vi "Start Print.vi"(8 "error in (no error)":errorcluster, 11 "Feeder Actor.lvlib:Feeder.lvclass":refnum<class "Feeder.lvclass">) -> (0 "error out":errorcluster, 3 "Feeder Actor.lvlib:Feeder.lvclass":refnum<class "Feeder.lvclass">)   [LabVIEW 2018, in "Feeder Actor.lvlib" / "Feeder.lvclass"]
uses:
  Feeder.lvclass
  Feeder.lvclass/Feeder.ctl
  Solenoid Messages/Set Solonoid Msg/Set Solonoid Msg.lvclass/Set Solonoid Msg.ctl
  <vilib>/ActorFramework/Message Enqueuer/Message Enqueuer.lvclass/Message Enqueuer.ctl
  <vilib>/ActorFramework/Message Enqueuer/Enqueue.vi
  Solenoid Messages/Set Solonoid Msg/Set Solonoid Msg.lvclass
  C:/Program Files/National Instruments/LabVIEW 2018/vi.lib/ActorFramework/Message/Message.lvclass
  <vilib>/ActorFramework/Message Priority Queue/Priority Enqueue.vi
  Mixer Messages/Mixer Print Msg/Mixer Print Msg.lvclass
  Screw Messages/Screw Print Msg/Screw Print Msg.lvclass
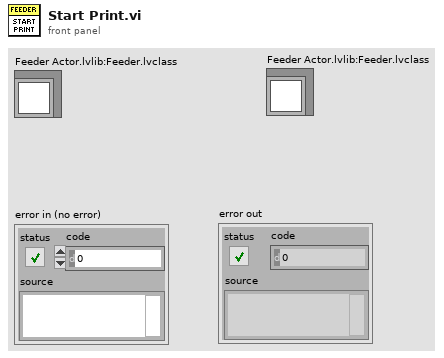
[diagram p1: front panel]
types:
  T1 = enum8{"Enabled", "Disabled", "Disabled and Grayed Out"}
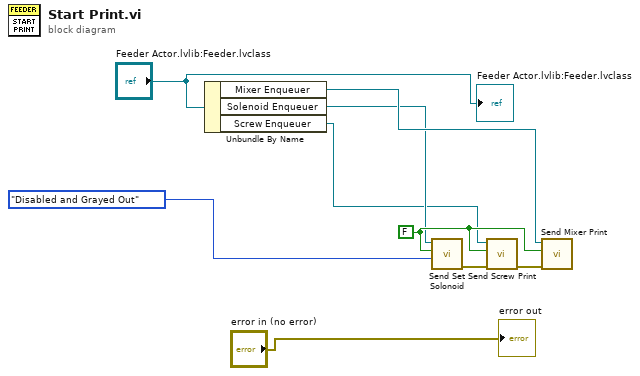
[diagram p0: block diagram]
diagram:
  w5 = FALSE ("State")
  n1 = Unbundle By Name("Feeder Actor.lvlib:Feeder.lvclass") -> ("Mixer Enqueuer"=w4:refnum<class "Message Enqueuer.lvclass">, "Solenoid Enqueuer"=w3:refnum<class "Message Enqueuer.lvclass">, "Screw Enqueuer"=w2:refnum<class "Message Enqueuer.lvclass">)
  n2 = call "Send Set Solonoid.vi"("Enabled?"=T1."Disabled and Grayed Out", "State"=w5, "Message Enqueuer in"=w3) -> ("error out"=w7:errorcluster)  [unwired: 7 in, 1 out]
  n3 = call "Send Screw Print.vi"("error in (no error)"=w7, "On?"=w5, "Message Enqueuer in"=w2) -> ("error out"=w6:errorcluster)  [unwired: 7 in, 1 out]
  n4 = call "Send Mixer Print.vi"("error in (no error)"=w6, "On?"=w5, "Message Enqueuer in"=w4) -> ()  [unwired: 7 in, 2 out]
  "Feeder Actor.lvlib:Feeder.lvclass" <- "Feeder Actor.lvlib:Feeder.lvclass"
  "error out" <- "error in (no error)"
